vi "is a.vi"(8 "error in (no error)":errorcluster, 11 "Cooling System in":refnum<class "Cooling System.lvclass">) -> (0 "error out":errorcluster, 2 "is a":string, 3 "Cooling System out":refnum<class "Cooling System.lvclass">)   [LabVIEW 2016, in "Hardware.lvlib" / "Cooling System.lvclass"]
uses:
  Cooling System.lvclass
  Hardware.lvclass
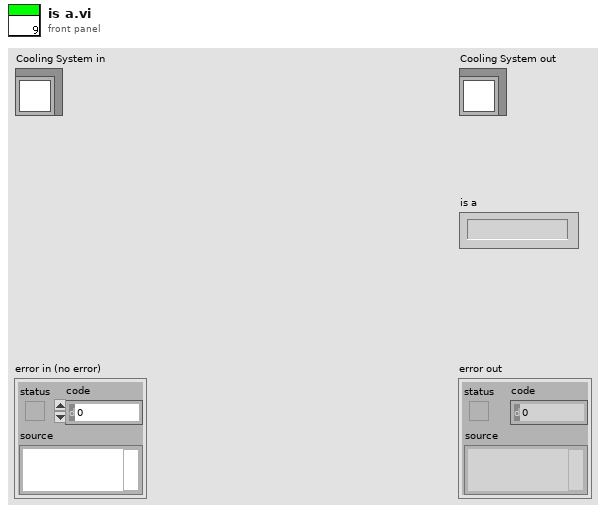
[diagram p1: front panel]
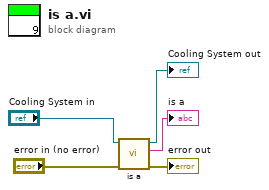
[diagram p0: block diagram]
diagram:
  n1 = call-parent "is a.vi"("error in (no error)"="error in (no error)", "Hardware in"="Cooling System in") -> ("error out"=→"error out":errorcluster, "is a"=→"is a":string, "Hardware out"=→"Cooling System out":refnum<class "Cooling System.lvclass">)  [unwired: 7 in]
